vi "testBooleanStringTrue.vi"(8 "error in (no error)":errorcluster, 11 "TestCase in":refnum<class "Python Data Tools Tests.lvclass">) -> (0 "error out":errorcluster, 3 "TestCase out":refnum<class "Python Data Tools Tests.lvclass">)   [LabVIEW 2020, in "Python Data Tools Tests.lvclass"]
uses:
  Python Data Tools Tests.lvclass
  Python Data Tools Tests.lvclass/Python Data Tools Tests.ctl
  <vilib>/addons/_JKI Toolkits/VI Tester/TestCase.llb/TestCase.lvclass
  source/jki_python_data_tools.lvlib
  C:/Program Files/National Instruments/LabVIEW 2020/vi.lib/addons/_JKI Toolkits/VI Tester/TestCase.llb/TestCase.lvclass
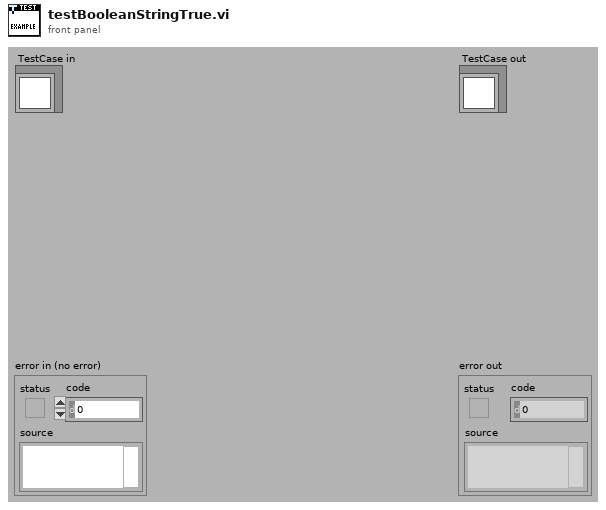
[diagram p1: front panel]
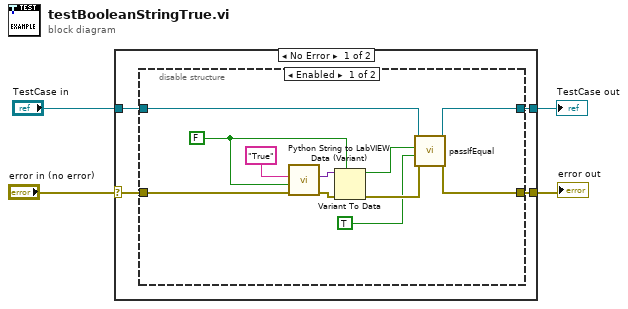
[diagram p0: block diagram]
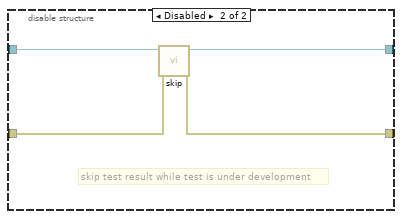
[diagram p2: hidden frame]
diagram:
  n1 = case shown="No Error" "error in (no error)" {
    selector: "error in (no error)" -> [w6 w25]
    tunnel: [w5 w25] -> w3
    tunnel: [w7 w24] -> w1
    tunnel: "TestCase in" -> [w8 w24]
    frame No Error {
      n2 = disable-structure shown="Enabled" {
        disable-tunnel: w8 -> [w19 w23]
        disable-tunnel: [w18 w20] -> w7
        disable-tunnel: w6 -> [w11 w22]
        disable-tunnel: [w17 w21] -> w5
        frame Enabled {
          w13 = FALSE
          n3 = call "Python String to LabVIEW Data (Variant).vi"("error in (no error)"=w11, "type"=w13, "Python String"="True") -> ("error out"=w15:errorcluster, "LabVIEW Data"=w16:variant)  [unwired: 7 in]
          n4 = Variant To Data(error in=w15, type=w13, Variant=w16) -> (data=w10:bool, error out=w14:errorcluster)
          n5 = call-dynamic "passIfEqual.vi"("error in (no error)"=w14, "y"=TRUE, "x"=w10, "TestCase in"=w19) -> ("error out"=w17:errorcluster, "TestCase out"=w18:refnum<class "Python Data Tools Tests.lvclass">)  [unwired: 6 in]
        }
        frame Disabled {
          # "skip test result while test is under development"
          n6 = call <vilib>:"skip.vi"("error in (no error)"=w22, "TestCase in"=w23) -> ("error out"=w21:errorcluster, "TestCase out"=w20:refnum<class "Python Data Tools Tests.lvclass">)  [unwired: 8 in]
        }
      }
    }
    frame Error {
    }
  }
  "error out" <- w3
  "TestCase out" <- w1
